vi "总氮版本号读取.vi"(8 "Error in":errorcluster caption="Error in (no error)") -> (0 "error out":errorcluster, 3 "固件版本号":string)   [LabVIEW 2016, in "总氮.lvlib"]
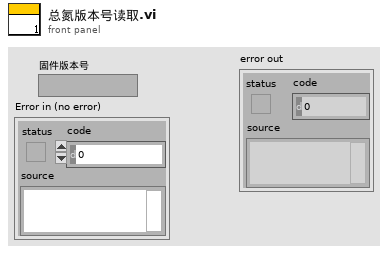
[diagram p1: front panel]
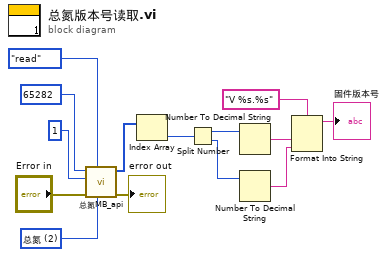
[diagram p0: block diagram]
diagram:
  w1 = u16 2 items=["总磷"=1, "总氮"=2, "氨氮"=3] ("站号")
  n1 = call "总氮MB_api.vi"("Slave ID"=w1, "STEP"=enum16{"open", "read", "write", "close"}."read", "Error in"="Error in", "quantity"=u16 1, "starting address"=u16 65282) -> ("error out"=→"error out":errorcluster, "Registers"=w11:u16[])  [unwired: 3 in, 2 out]
  n2 = Index Array(array=w11) -> (element=w10:u16)  [unwired: 1 in]
  n3 = Split Number(x=w10) -> (hi(x)=w9:u8, lo(x)=w8:u8)
  n4 = Number To Decimal String(number=w9) -> (decimal integer string=w7:string)  [unwired: 1 in]
  n5 = Number To Decimal String(number=w8) -> (decimal integer string=w6:string)  [unwired: 1 in]
  n6 = Format Into String(format string="V %s.%s" ("格式字符串"), w7, w6) -> (resulting string=→"固件版本号":string)  [unwired: 2 in, 1 out]
